vi "ActionVIOnCompile.vi"(8 "error in (no error)":errorcluster, 11 "Device Item Ref in":T1 format="%.0x") -> (0 "error out":errorcluster)   [LabVIEW 2020, in "PXI-2510 System Explorer.lvlib"]
uses:
  PXI-2510 System Explorer.lvlib
  <vilib>/NI VeriStand/Custom Device API/Custom Device Item Ref.ctl
  Shared/Compiled.Settings.ctl
  Shared/Constants.vi
  <vilib>/NI VeriStand/Custom Device Tools/Custom Device Utility Library/NI VeriStand - Search for Item by Name.vi
  <vilib>/NI VeriStand/Custom Device API/Set Item Property (Variant).vi
  <vilib>/NI VeriStand/Custom Device API/Get Item Property (String).vi
  <vilib>/NI VeriStand/Custom Device API/Get Item Property (U16).vi
  <vilib>/NI VeriStand/Custom Device Tools/Custom Device Utility Library/Custom Device Utility Library.lvlib
  <vilib>/NI VeriStand/Custom Device API/Custom Device API.lvlib
  <vilib>/NI/NIVS Inline Async API/_Data Access System Explorer/Data Access System Explorer.lvlib
  Shared/PXI-2510 Shared.lvlib
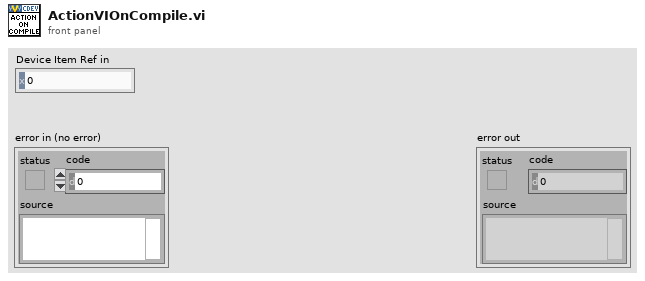
[diagram p1: front panel]
types:
  T1 = typedef "Custom Device API.lvlib/Custom Device Item Ref.ctl" = u64
  T2 = cluster{"Name":string, "Type":enum16{"Output/Write", "Input/Read", "Input/ReadWrite"}, "VS Refs":T1[]}
  T3 = enum16{"Output/Write", "Input/Read", "Input/ReadWrite"}
  T4 = typedef "PXI-2510 Shared.lvlib/Compiled.Settings.ctl" = cluster{"Name":string, "Async Init Timeout":u16, "Hardware Device Name":string}
  T5 = typedef "Custom Device API.lvlib/Custom Device Item Info.ctl" = cluster{"Name":string, "Is Channel":bool, "GUID":string, "Is Waveform":bool}
  T6 = cluster{"Name":string, "Type":enum16{"Output/Write", "Input/Read", "Input/ReadWrite"}, "VS Refs":T1[]}[]
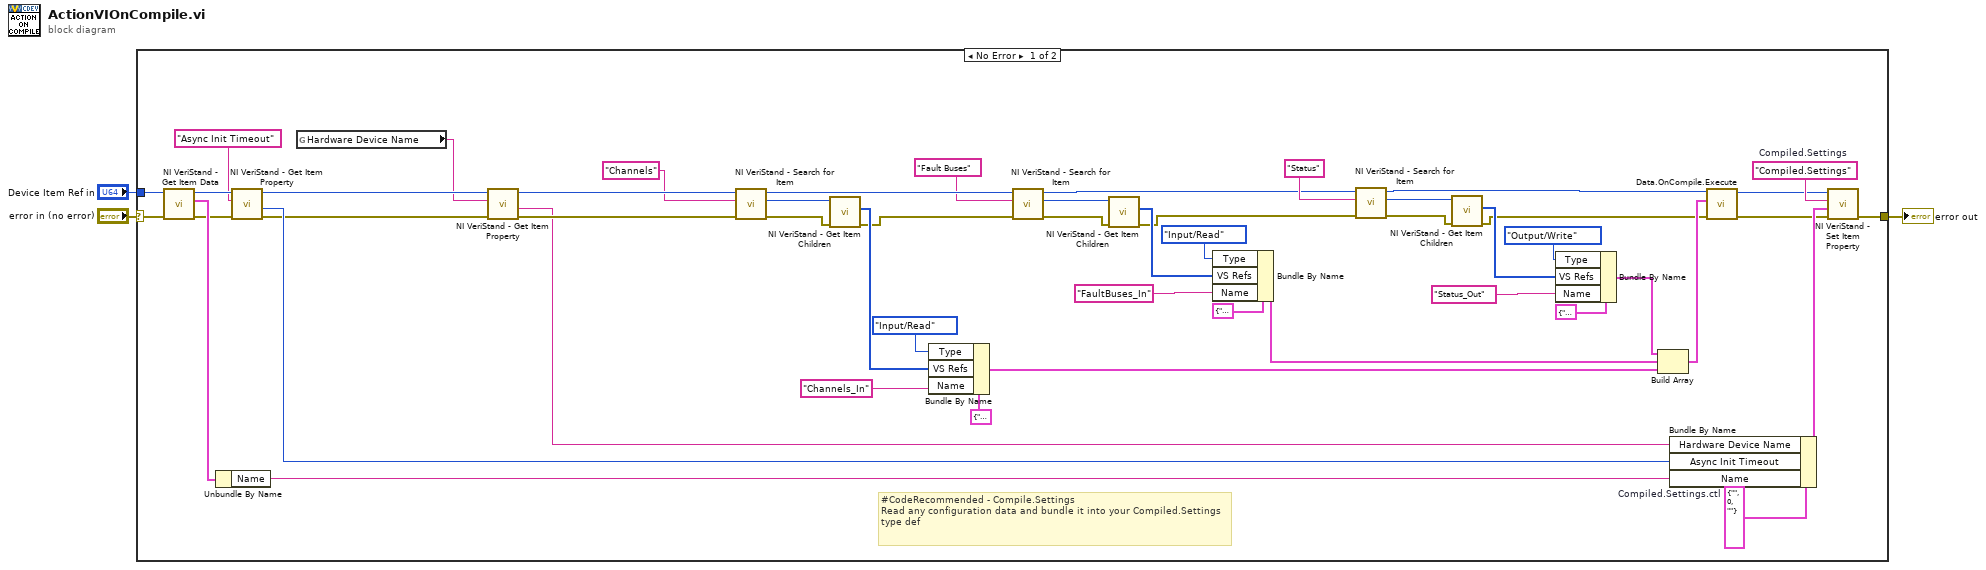
[diagram p0: block diagram]
diagram:
  n1 = case shown="No Error" "error in (no error)" {
    selector: "error in (no error)" -> [w47 w55]
    tunnel: [w48 w55] -> w2
    tunnel: "Device Item Ref in" -> [w46 _]
    frame No Error {
      w29 = T4 {"Name"="", "Async Init Timeout"=0, "Hardware Device Name"=""}  # Compiled.Settings.ctl
      w50 = "Compiled.Settings"  # Compiled.Settings
      # "#CodeRecommended - Compile.Settings\nRead any configuration data and bundle it into your Compiled.Settings type def"
      n2 = call <vilib>:"NI VeriStand - Get Item Data.vi"("error in (no error)"=w47, "Item Ref in"=w46) -> ("error out"=w28:errorcluster, "Item Info"=w45:T5, "Item Ref out"=w27:T1)  [unwired: 6 in, 1 out]
      n3 = Unbundle By Name(w45) -> ("Name"=w44:string)
      n4 = call-poly <vilib>:"NI VeriStand - Get Item Property.vi"("error in (no error)"=w28, "Property Name"="Async Init Timeout", "Item Ref in"=w27) -> ("error out"=w22:errorcluster, "Value"=w25:u16, "Item Ref out"=w24:T1)  [unwired: 5 in, 1 out]
      n5 = global read "Constants.vi" "Hardware Device Name"() -> (w20:string)
      n6 = call-poly <vilib>:"NI VeriStand - Get Item Property.vi"("error in (no error)"=w22, "Property Name"=w20, "Item Ref in"=w24) -> ("error out"=w21:errorcluster, "Value"=w19:string, "Item Ref out"=w23:T1)  [unwired: 5 in, 1 out]
      n7 = call-poly <vilib>:"NI VeriStand - Search for Item.vi"("error in"=w21, "Item Name"="Channels", "Section Ref in"=w23) -> ("error out"=w54:errorcluster, "Item Ref"=w53:T1, "Section Ref out"=w33:T1)  [unwired: 5 in, 1 out]
      n8 = call <vilib>:"NI VeriStand - Get Item Children.vi"("error in (no error)"=w54, "Item Ref in"=w53) -> ("error out"=w32:errorcluster, "Child Refs"=w43:T1[])  [unwired: 6 in, 2 out]
      n9 = Bundle By Name(cluster=T2 {"Name"="", "Type"=enum."Output/Write", "VS Refs"=[]} ("Group"), "Type"=T3."Input/Read", "VS Refs"=w43, "Name"="Channels_In" ("Item Name")) -> (w34:T2)
      n10 = call-poly <vilib>:"NI VeriStand - Search for Item.vi"("error in"=w32, "Item Name"="Fault Buses", "Section Ref in"=w33) -> ("error out"=w51:errorcluster, "Item Ref"=w52:T1, "Section Ref out"=w7:T1)  [unwired: 5 in, 1 out]
      n11 = call <vilib>:"NI VeriStand - Get Item Children.vi"("error in (no error)"=w51, "Item Ref in"=w52) -> ("error out"=w8:errorcluster, "Child Refs"=w38:T1[])  [unwired: 6 in, 2 out]
      n12 = Bundle By Name(cluster=T2 {"Name"="", "Type"=enum."Output/Write", "VS Refs"=[]} ("Group"), "Type"=T3."Input/Read", "VS Refs"=w38, "Name"="FaultBuses_In" ("Item Name")) -> (w40:T2)
      n13 = call-poly <vilib>:"NI VeriStand - Search for Item.vi"("error in"=w8, "Item Name"="Status", "Section Ref in"=w7) -> ("error out"=w14:errorcluster, "Item Ref"=w15:T1, "Section Ref out"=w5:T1)  [unwired: 5 in, 1 out]
      n14 = call <vilib>:"NI VeriStand - Get Item Children.vi"("error in (no error)"=w14, "Item Ref in"=w15) -> ("error out"=w6:errorcluster, "Child Refs"=w11:T1[])  [unwired: 6 in, 2 out]
      n15 = Bundle By Name(cluster=T2 {"Name"="", "Type"=enum."Output/Write", "VS Refs"=[]} ("Group"), "Type"=T3."Output/Write", "VS Refs"=w11, "Name"="Status_Out" ("Item Name")) -> (w4:T2)
      n16 = Build Array(w4, w40, w34) -> (w37:T6)
      n17 = Bundle By Name(cluster=w29, "Hardware Device Name"=w19, "Async Init Timeout"=w25, "Name"=w44) -> (w49:T4)
      n18 = call <vilib>:"Data.OnCompile.Execute.vi"("error in"=w6, "VS Ref Groups"=w37, "Custom Device Ref"=w5) -> ("error out"=w31:errorcluster, "Custom Device Ref"=w30:T1)  [unwired: 7 in]
      n19 = call-poly <vilib>:"NI VeriStand - Set Item Property.vi"("error in (no error)"=w31, "Value"=w49, "Property Name"=w50, "Item Ref in"=w30) -> ("error out"=w48:errorcluster)  [unwired: 5 in, 2 out]
    }
    frame Error {
    }
  }
  "error out" <- w2
